vi "itc box.vi"() -> ()   [LabVIEW 2010]
panel:
  in  "action":T1(ring)
  out "error out":errorcluster
  out "ITC503 Address out":refnum<visa-resource-name>
  in  "ITC503 Address":refnum<visa-resource-name>
  in  "error in":errorcluster
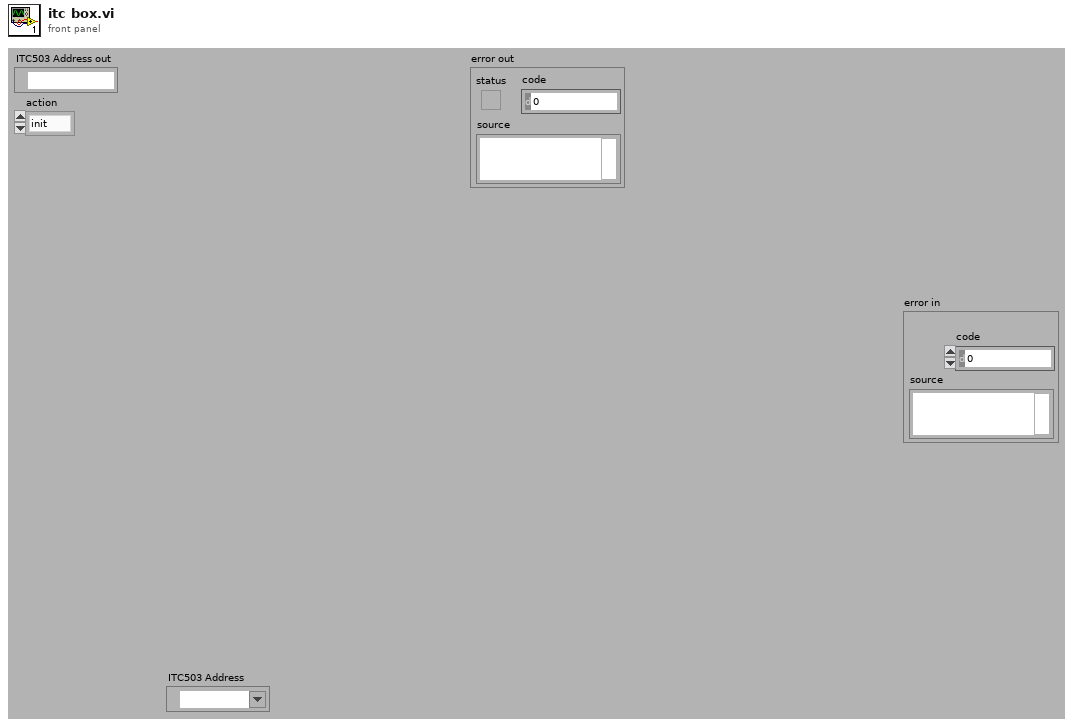
[diagram p1: front panel]
types:
  T1 = enum16{"init", "start sweep", "stop sweep", "heater auto", "heater manual", "set heater"}
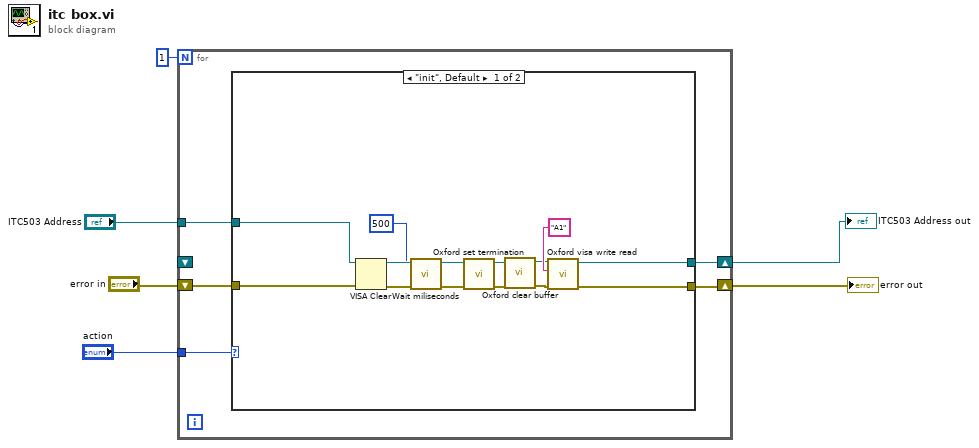
[diagram p0: block diagram]
diagram:
  n1 = for {
    N: 1 -> [_]
    shift-right: [w11] -> w5
    shift-left: _ -> [_]
    shift-right: [w9] -> w3
    shift-left: "error in" -> [w10]
    tunnel: "ITC503 Address" -> [w8]
    tunnel: "action" -> [w7]
    n2 = case shown="\"init\", Default" w7 {
      tunnel: [w15 _] -> w11
      tunnel: w10 -> [w14 _]
      tunnel: [w13 _] -> w9
      tunnel: w8 -> [w12 _]
      frame "init", Default {
        n3 = VISA Clear(VISA resource name=w12, error in (no error)=w14) -> (VISA resource name out=w24:refnum<visa-resource-name>, error out=w18:errorcluster)
        n4 = call "Wait miliseconds.vi"("error in (no error)"=w18, "milliseconds to wait"=u32 500) -> ("error out"=w17:errorcluster)  [unwired: 8 in, 1 out]
        n5 = call "Oxford set termination.vi"("error in (no error)"=w17, "VISA resource name"=w24) -> ("error out"=w22:errorcluster, "VISA resource name out"=w20:refnum<visa-resource-name>)  [unwired: 8 in]
        n6 = call "Oxford clear buffer.vi"("error in (no error)"=w22, "VISA resource name"=w20) -> ("error out"=w21:errorcluster, "VISA resource name out"=w19:refnum<visa-resource-name>)  [unwired: 6 in, 2 out]
        n7 = call "Oxford visa write read.vi"("error in (no error)"=w21, "write buffer"="A1" ("Command"), "VISA resource name"=w19) -> ("error out"=w13:errorcluster, "VISA resource name out"=w15:refnum<visa-resource-name>)  [unwired: 6 in, 1 out]
      }
      frame "start sweep" {
      }
    }
  }
  "ITC503 Address out" <- w5
  "error out" <- w3
